vi "TB-Init Mic Queue.vi"(0 "state in":T4, 9 "Number":i32, 11 "error in (no error)":errorcluster, 13 "Pistonphone factor":dbl, 14 "Exposure parameters":T1={"Low cutoff (kHz)"=0.0, "High cutoff (kHz)"=0.0, "Duration (min)"=0.0, "dB SPL"=100.0, "Waveform"=enum."Noise", "WAVfile"=path "", "refWav"=path "", "use mic correction"=FALSE, "micCorrFile"=path "", "Pistonphone Level (dB SPL)"=0.0, "Sampling rate (Hz)"=0.0, "Buffer length (s)"=0.0, "Stream mic"=FALSE, "Fine adjust"={"Max"=0.0, "Min"=0.0}, "Mic gain"=0.0, "atten"=0.0, "Allow Slack"=FALSE, "max starts"=0, "Freq (kHz)"=8.0, "Tma (s)"=0.0, "Streamed"=[], "Drive"="", "Speaker"="", "Mic"="", "Analysis"={"Method"=enum."Default", "resol (Hz)"=0.0, "nfreq"=0, "signal"=""}}) -> (4 "state out":T4, 6 "mic queue":T3, 15 "error out":errorcluster)   [LabVIEW 2020]
uses:
  Typedefs/TB-Runtime state.ctl
  <vilib>/sound2/lvsound2.llb/Sound File Refnum.ctl
  Typedefs/TB-Setup Log.ctl
  Typedefs/TB-Analysis State.ctl
  Typedefs/TB-Mic Queue.ctl
  Typedefs/TB-Parameters.ctl
  Typedefs/TB-Analysis Parameters.ctl
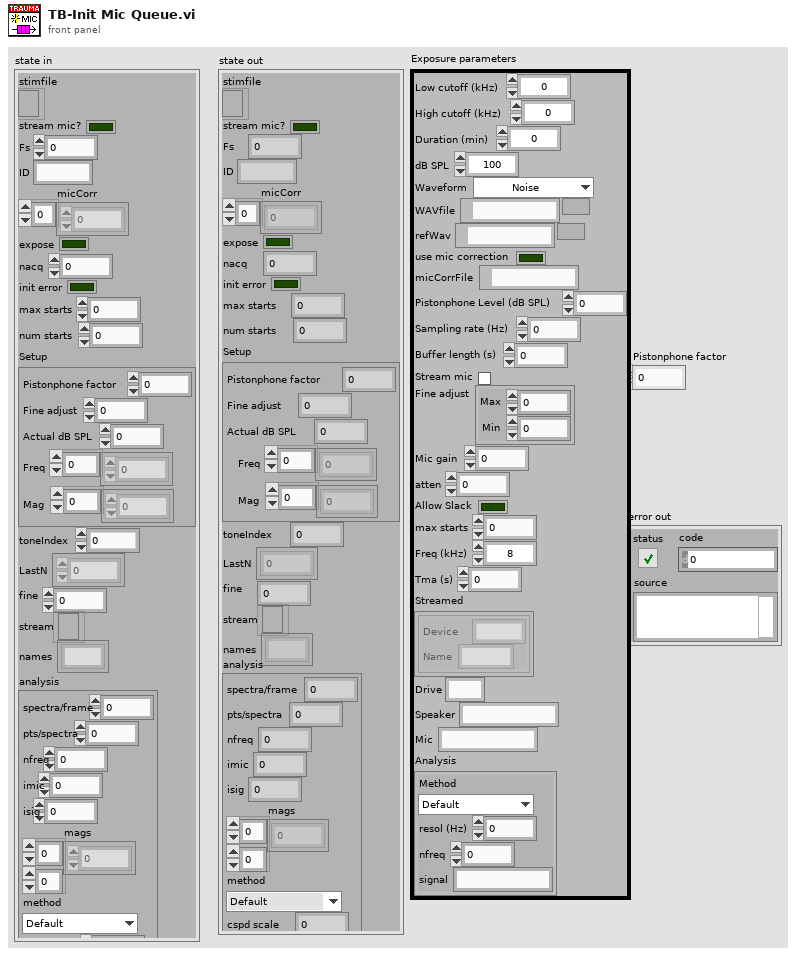
[diagram p1: front panel]
types:
  T1 = typedef "TB-Parameters.ctl" = cluster{"Low cutoff (kHz)":dbl, "High cutoff (kHz)":dbl, "Duration (min)":dbl, "dB SPL":dbl, "Waveform":enum16{"Noise", "File", "Tone"}, "WAVfile":path, "refWav":path, "use mic correction":bool, "micCorrFile":path, "Pistonphone Level (dB SPL)":dbl, "Sampling rate (Hz)":dbl, "Buffer length (s)":dbl, "Stream mic":bool, "Fine adjust":cluster{"Max":dbl, "Min":dbl}, "Mic gain":dbl, "atten":dbl, "Allow Slack":bool, "max starts":i32, "Freq (kHz)":dbl, "Tma (s)":dbl, "Streamed":cluster{"Device":string, "Name":string}[], "Drive":string, "Speaker":string, "Mic":string, "Analysis":T2}
  T2 = typedef "TB-Analysis Parameters.ctl" = cluster{"Method":enum16{"Default", "Periodogram", "Cross-spectrum"}, "resol (Hz)":dbl, "nfreq":i32, "signal":string}
  T3 = typedef "TB-Mic Queue.ctl" = refnum<queue>
  T4 = typedef "TB-Runtime state.ctl" = cluster{"stimfile":T5, "stream mic?":bool, "Fs":dbl, "ID":string, "micCorr":dbl[], "expose":bool, "nacq":i32, "init error":bool, "max starts":i32, "num starts":i32, "Setup":T6, "toneIndex":i32, "LastN":dbl[], "fine":dbl, "stream":refnum<file>, "names":string[], "analysis":T7}
  T5 = typedef "Sound File Refnum.ctl" = refnum<file>
  T6 = typedef "TB-Setup Log.ctl" = cluster{"Pistonphone factor":dbl, "Fine adjust":dbl, "Actual dB SPL":dbl, "Freq":dbl[], "Mag":dbl[]}
  T7 = typedef "TB-Analysis State.ctl" = cluster{"spectra/frame":i32, "pts/spectra":i32, "nfreq":i32, "imic":i32, "isig":i32, "mags":dbl[][], "method":enum16{"Default", "Periodogram", "Cross-spectrum"}, "cspd scale":dbl}
  T8 = enum16{"open", "replace", "create", "open or create", "replace or create", "replace or create with confirmation"}
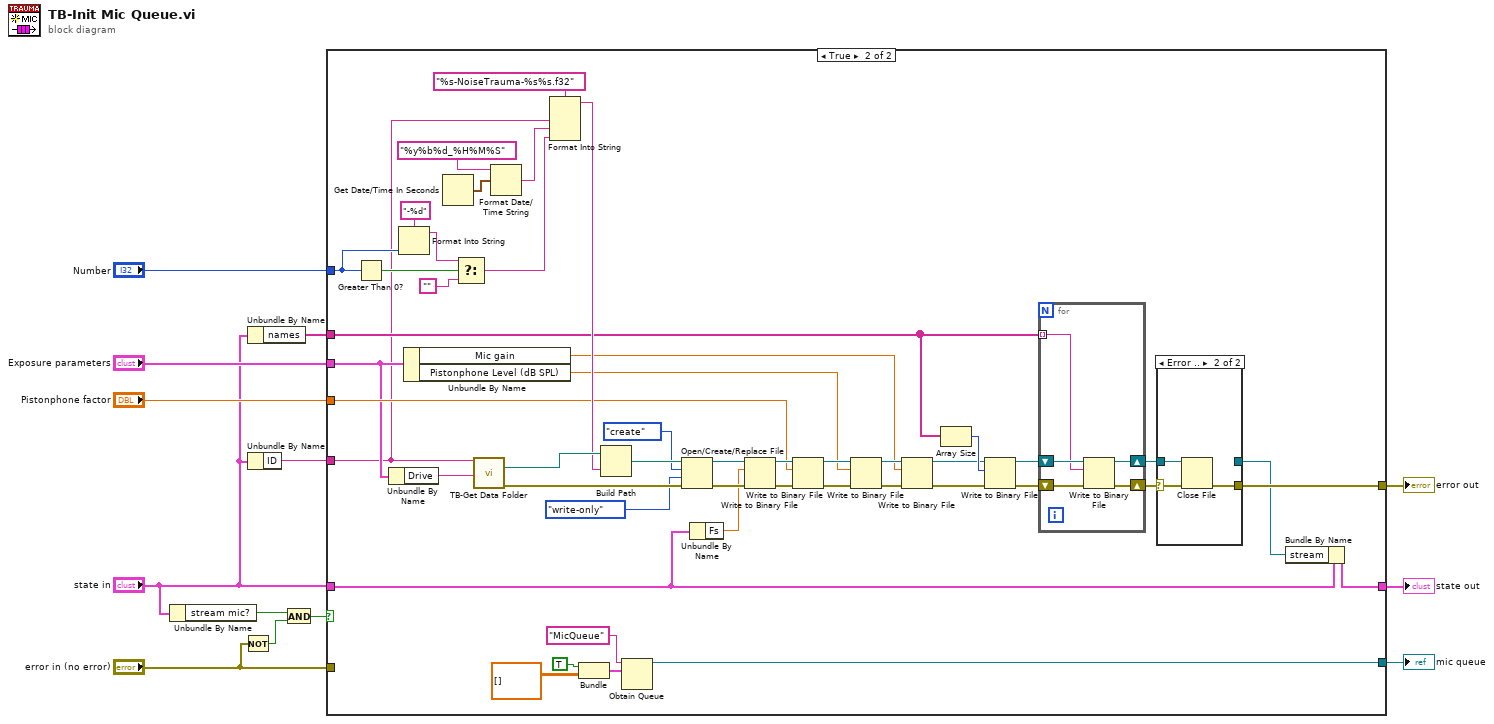
[diagram p0: block diagram]
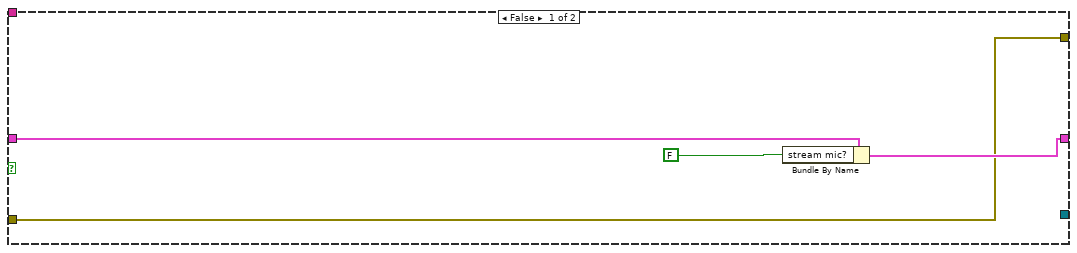
[diagram p2: hidden frame]
diagram:
  n1 = Unbundle By Name("state in") -> ("stream mic?"=w12:bool)
  n2 = Not(x="error in (no error)") -> (.not. x?=w13:bool)
  n3 = Unbundle By Name("state in") -> ("names"=w1:string[])
  n4 = Unbundle By Name("state in") -> ("ID"=w8:string)
  n5 = And(x=w12, y=w13) -> (x .and. y?=w10:bool)
  n6 = case shown="True" w10 {
    tunnel: [w16 w64] -> w7
    tunnel: "state in" -> [w17 w65]
    tunnel: w8 -> [_ w18]
    tunnel: [_ w53] -> w11
    tunnel: "error in (no error)" -> [w14 _]
    tunnel: "Number" -> [_ w47]
    tunnel: w1 -> [_ w36]
    tunnel: [w14 w33] -> w5
    tunnel: "Pistonphone factor" -> [_ w29]
    tunnel: "Exposure parameters" -> [_ w20]
    frame False {
      n7 = Bundle By Name(cluster=w17, "stream mic?"=FALSE ("micfile?")) -> (w16:T4)
    }
    frame True {
      n8 = Greater Than 0?(x=w47) -> (x > 0?=w51:bool)
      n9 = Unbundle By Name(w20) -> ("Drive"=w19:string)
      n10 = Format Into String(format string="-%d", w47) -> (resulting string=w48:string)  [unwired: 2 in, 1 out]
      n11 = Unbundle By Name(w20) -> ("Mic gain"=w22:dbl, "Pistonphone Level (dB SPL)"=w21:dbl)
      n12 = Get Date/Time In Seconds() -> (seconds since 1Jan1904=w60:timestamp)
      n13 = Select(t=w48, s=w51, f="") -> (s? t:f=w49:string)
      n14 = call "TB-Get Data Folder.vi"("ID"=w18, "Drive"=w19) -> ("Data folder"=w63:path, "error out"=w45:errorcluster)  [unwired: 12 in]
      n15 = Format Date/Time String(time format string (%c)="%y%b%d_%H%M%S", seconds (now)=w60) -> (date/time string=w58:string)  [unwired: 1 in]
      n16 = Format Into String(format string="%s-NoiseTrauma-%s%s.f32", w18, w58, w49) -> (resulting string=w61:string)  [unwired: 2 in, 1 out]
      n17 = Bundle(TRUE, dbl[][] []) -> (w56:cluster{bool, dbl[][]})  [unwired: 1 in]
      n18 = Build Path(base path=w63, name or relative path=w61) -> (appended path=w46:path)
      n19 = Obtain Queue(name (unnamed)="MicQueue", element data type=w56) -> (queue out=w53:refnum<queue>)  [unwired: 3 in, 2 out]
      n20 = Open/Create/Replace File(file path (use dialog)=w46, error in=w45, operation (0:open)=T8."create", access (0:read/write)=enum16{"read/write", "read-only", "write-only"}."write-only") -> (refnum out=w41:refnum<file>, error out=w42:errorcluster)  [unwired: 2 in, 1 out]
      n21 = Unbundle By Name(w65) -> ("Fs"=w40:dbl)
      n22 = Write to Binary File(file (use dialog)=w41, data=w40, error in=w42) -> (refnum out=w30:refnum<file>, error out=w31:errorcluster)  [unwired: 3 in, 1 out]
      n23 = Write to Binary File(file (use dialog)=w30, data=w29, error in=w31) -> (refnum out=w27:refnum<file>, error out=w28:errorcluster)  [unwired: 3 in, 1 out]
      n24 = Write to Binary File(file (use dialog)=w27, data=w21, error in=w28) -> (refnum out=w25:refnum<file>, error out=w26:errorcluster)  [unwired: 3 in, 1 out]
      n25 = Write to Binary File(file (use dialog)=w25, data=w22, error in=w26) -> (refnum out=w24:refnum<file>, error out=w23:errorcluster)  [unwired: 3 in, 1 out]
      n26 = Array Size(array=w36) -> (size(s)=w39:i32)
      n27 = Write to Binary File(file (use dialog)=w24, data=w39, error in=w23) -> (refnum out=w37:refnum<file>, error out=w38:errorcluster)  [unwired: 3 in, 1 out]
      n28 = for {
        shift-right: [w69] -> w35
        shift-left: w38 -> [w70]
        shift-right: [w67] -> w34
        shift-left: w37 -> [w68]
        tunnel: w36 -> [w66] mode=indexing
        n29 = Write to Binary File(file (use dialog)=w68, data=w66, error in=w70) -> (refnum out=w67:refnum<file>, error out=w69:errorcluster)  [unwired: 3 in, 1 out]
      }
      n30 = case shown="Error .." w35 {
        selector: w35 -> [w72 w75]
        tunnel: w34 -> [w71 w74]
        tunnel: [w72 w73] -> w33
        tunnel: [w71 _] -> w32
        frame No Error {
        }
        frame Error {
          n31 = Close File(refnum=w74, error in=w75) -> (error out=w73:errorcluster)  [unwired: 1 out]
        }
      }
      n32 = Bundle By Name(cluster=w65, "stream"=w32) -> (w64:T4)
    }
  }
  "error out" <- w5
  "state out" <- w7
  "mic queue" <- w11
